vi "TaskFor_P3ATRTdata_Message.vi"(8 "error in (no error)":errorcluster caption="错误输入（无错误）", 10 "P3AT_RT_data":T1, 11 "MapDisplayer输入":refnum<class "MapDisplayer.lvclass">) -> (0 "error out":errorcluster caption="错误输出", 3 "MapDisplayer输出":refnum<class "MapDisplayer.lvclass">)   [LabVIEW 2014]
uses:
  MapDisplayer.lvclass
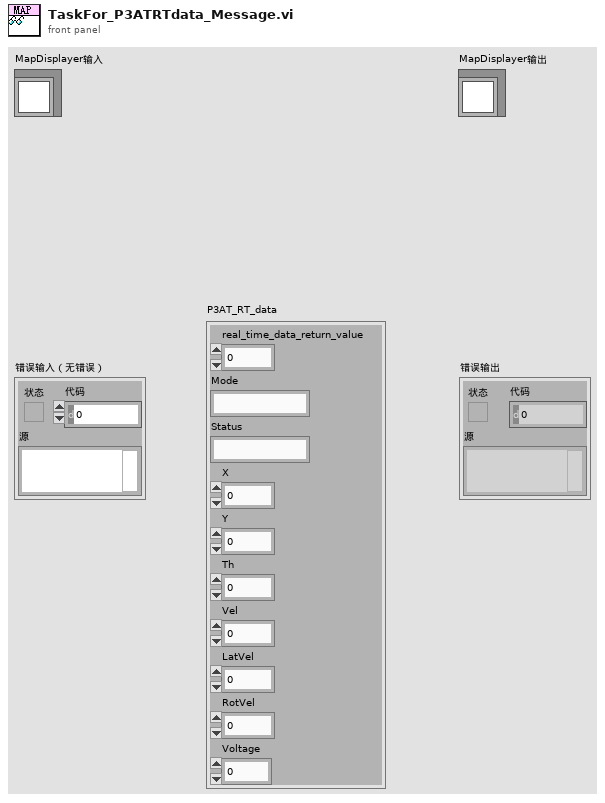
[diagram p1: front panel]
types:
  T1 = cluster{"real_time_data_return_value":i32, "Mode":string, "Status":string, "X":dbl, "Y":dbl, "Th":dbl, "Vel":dbl, "LatVel":dbl, "RotVel":dbl, "Voltage":dbl}
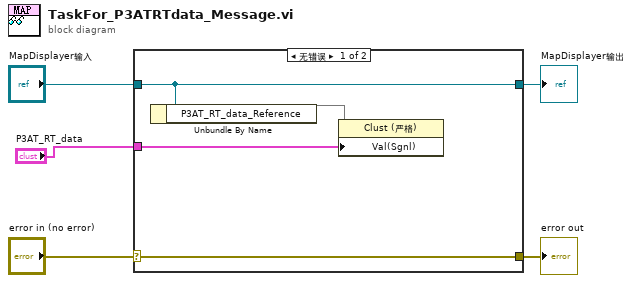
[diagram p0: block diagram]
diagram:
  n1 = case shown="无错误" "error in (no error)" {
    selector: "error in (no error)" -> [w9 w10]
    tunnel: [w9 w10] -> w4
    tunnel: [w8 w11] -> w2
    tunnel: "MapDisplayer输入" -> [w8 w11]
    tunnel: "P3AT_RT_data" -> [w6 _]
    frame No Error {
      n2 = Unbundle By Name(w8) -> ("P3AT_RT_data_Reference"=w7)
      n3 = property class="Clust (严格)"(reference=w7, "Val(Sgnl)"=w6) -> ()  [unwired: 1 in, 2 out]
    }
    frame Error {
    }
  }
  "error out" <- w4
  "MapDisplayer输出" <- w2
